vi "Balik.vi"   [LabVIEW 2016, in "Test.lvrbt"]
uses:
  Test.lvrbt
  <vilib>/NXT/Hardware/Plugins/Tetrix DC Motor/TetrixDCMotorAddress.ctl
  <vilib>/NXT/NXTIO Xnodes/NXTIONodeSubVIs/TETRIX IO Move DC Motors.vi
  <vilib>/NXT/Dual Mode Library/Waits/Wait_Num.vi
  <vilib>/NXT/NXTIO Xnodes/NXTIONodeSubVIs/TETRIX IO Stop DC Motors.vi
  <vilib>/NXT/Subs/LVHSConnector.ctl
  <vilib>/NXT/NXTIO Xnodes/AddressXNode/NXTIOAddress.xnode
  <vilib>/NXT/NXTIO Xnodes/NXTIOXNode/NXTIO.xnode
  <vilib>/NXT/LegoClasses/BrickReference/BrickReference.lvclass
types:
  T1 = typedef "TetrixDCMotorAddress.ctl" = i32
  T2 = typedef "LVHSConnector.ctl" = refnum<class "BrickReference.lvclass">
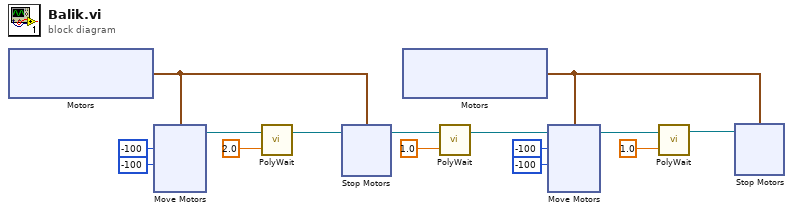
[diagram p0: block diagram]
diagram:
  n1 = xnode "Motors"() -> ("Motor"=w10:cluster{"TetrixDCMotor":T1, "TetrixDCMotor":T1})
  n2 = xnode "Move Motors"("Power/Speed 2"=i8 -100, "Power/Speed 1"=i8 -100, "Motors"=w10) -> ("NXT/EV3"=w13:T2)  [unwired: 1 in]
  n3 = call-poly <vilib>:"PolyWait.vi"("Time (1 sec)"=sgl 2.0, "NXT/EV3"=w13) -> ("NXT/EV3"=w11:T2)  [unwired: 2 in]
  n4 = xnode "Stop Motors"("Motors"=w10, "NXT/EV3"=w11) -> ("NXT/EV3"=w8:T2)
  n5 = xnode "Motors"() -> ("Motor"=w1:cluster{"TetrixDCMotor":T1, "TetrixDCMotor":T1})
  n6 = call-poly <vilib>:"PolyWait.vi"("Time (1 sec)"=sgl 1.0, "NXT/EV3"=w8) -> ("NXT/EV3"=w5:T2)  [unwired: 2 in]
  n7 = xnode "Move Motors"("Power/Speed 2"=i8 -100, "Power/Speed 1"=i8 -100, "Motors"=w1, "NXT/EV3"=w5) -> ("NXT/EV3"=w3:T2)
  n8 = call-poly <vilib>:"PolyWait.vi"("Time (1 sec)"=sgl 1.0, "NXT/EV3"=w3) -> ("NXT/EV3"=w2:T2)  [unwired: 2 in]
  n9 = xnode "Stop Motors"("Motors"=w1, "NXT/EV3"=w2) -> ()  [unwired: 1 out]
